vi "Queue Status.vi"(8 "error in (no error)":errorcluster, 11 "queue name in":string) -> (0 "error out":errorcluster, 3 "queue status":T2)   [LabVIEW 2020]
uses:
  Control/Queue Data.ctl
panel:
  in  "return elements? (F)":bool
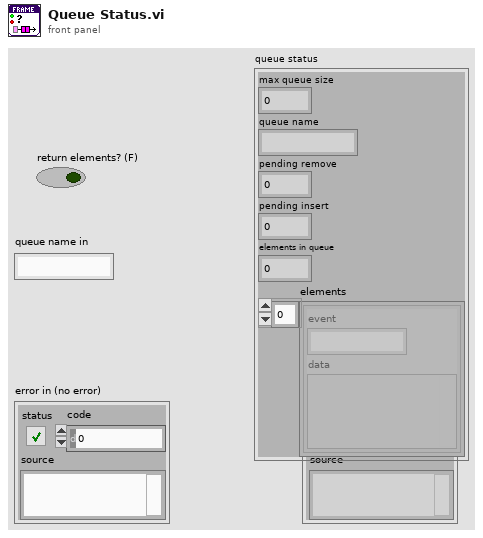
[diagram p1: front panel]
types:
  T1 = typedef "Queue Data.ctl" = cluster{"event":string, "data":variant}
  T2 = cluster{"max queue size":i32, "queue name":string, "pending remove":i32, "pending insert":i32, "elements in queue":i32, "elements":T1[]}
  T3 = cluster{"max queue size":i32, string, "# pending remove":i32, "# pending insert":i32, "# elements in queue":i32, "elements":T1[]}
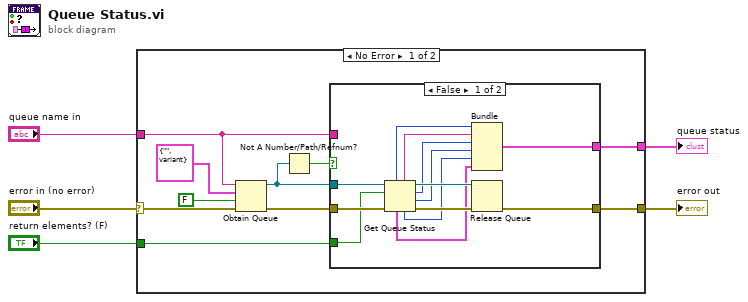
[diagram p0: block diagram]
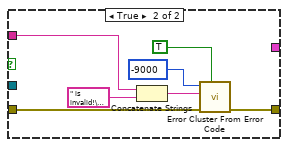
[diagram p2: hidden frame]
diagram:
  n1 = case shown="No Error" "error in (no error)" {
    selector: "error in (no error)" -> [w15 w36]
    tunnel: [w8 w36] -> w4
    tunnel: "queue name in" -> [w9 _]
    tunnel: "return elements? (F)" -> [w7 _]
    tunnel: [w6 _] -> w1
    frame No Error {
      n2 = Obtain Queue(name (unnamed)=w9, element data type=T1 {"event"="", "data"=variant}, create if not found? (T)=FALSE, error in (no error)=w15) -> (queue out=w11:refnum<queue>, error out=w12:errorcluster)  [unwired: 1 in, 1 out]
      n3 = Not A Number/Path/Refnum?(number/path/refnum=w11) -> (NaN/Path/Refnum?=w10:bool)
      n4 = case shown="False" w10 {
        tunnel: w12 -> [w27 w31]
        tunnel: w11 -> [w24 _]
        tunnel: w9 -> [_ w30]
        tunnel: [w28 w29] -> w8
        tunnel: w7 -> [w23 _]
        tunnel: [w16 _] -> w6
        frame False {
          n5 = Get Queue Status(queue=w24, return elements? (F)=w23, error in (no error)=w27) -> (queue out=w25:refnum<queue>, queue name=w21:string, max queue size=w22:i32, # pending remove=w20:i32, # pending insert=w19:i32, error out=w26:errorcluster, # elements in queue=w18:i32, elements=w17:T1[])
          n6 = Bundle("max queue size"=w22, w21, "# pending remove"=w20, "# pending insert"=w19, "# elements in queue"=w18, "elements"=w17) -> (w16:T3)  [unwired: 1 in]
          n7 = Release Queue(queue=w25, error in (no error)=w26) -> (error out=w28:errorcluster)  [unwired: 1 in, 2 out]
        }
        frame True {
          n8 = Concatenate Strings(w30, " is invalid!\nEnsure the queue has been created!" ("字符串")) -> (w35:string)
          n9 = call <vilib>:"Error Cluster From Error Code.vi"("show call chain? (False)"=TRUE, "error in (no error)"=w31, "error message (\"\")"=w35, "error code (0)"=-9000) -> ("error out"=w29:errorcluster)  [unwired: 5 in]
        }
      }
    }
    frame Error {
    }
  }
  "error out" <- w4
  "queue status" <- w1
